vi "fromDevVarCharArray.vi"(1 "argin":u8[](array[numeric])) -> (0 "ArgIO":cluster{"num data":u8[], "str data":string[]})   [LabVIEW 2014, in "tango.lvlib"]
uses:
  tango.lvlib
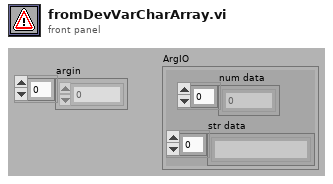
[diagram p1: front panel]
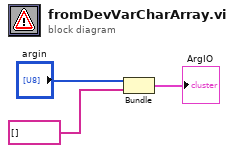
[diagram p0: block diagram]
diagram:
  n1 = Bundle("argin"="argin", string[] []) -> (→"ArgIO":cluster{"argin":u8[], string[]})  [unwired: 1 in]
